vi "graphics.vi"() -> ()   [LabVIEW 2018]
panel:
  in  "Tab Control":enum32{"CONTROLLER", "TEMP", "PRESSURE"}(tab)
  out "FEED WATER\nMOTOR AMPS\nPHASE A":dbl(knob) scale=0.0..10.0
  in  "V in":dbl
  out "Vout 2":dbl
  out "Vin":u8(slide) scale=0.0..100.0
  out "Vout":u8(slide) scale=0.0..20.0
  out "FEED WATER \nMOTOR AMPS \nPHASE B":dbl(knob) scale=0.0..10.0
  in  "DEG F":dbl
  out "DEG C":dbl
  out "DEG\nF":u8(slide) scale=0.0..100.0
  out "DEG\nC":u8(slide) scale=0.0..100.0
  out "FEED WATER \nMOTOR AMPS\nPHASE C":dbl(knob) scale=0.0..10.0
  in  "lbs/sq in":dbl
  out "mm Hg":dbl
  out "lb/sq\nin":u8(slide) scale=0.0..100.0
  out "mm\nHg":u8(slide) scale=0.0..100.0
  in  "stop":bool
  # "BOILER #1 FEED\nWATER CONTROL"
  # "FIC 1000\nFEED WATER\nCONTROLLER"
  # "FIC 1000\nFEED WATER\nTEMP"
  # "FIC 1000\nFEED WATER\nPRESSURE"
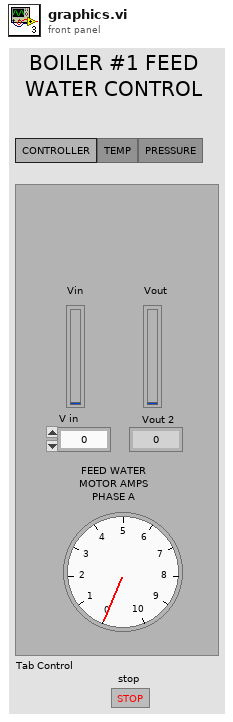
[diagram p1: front panel]
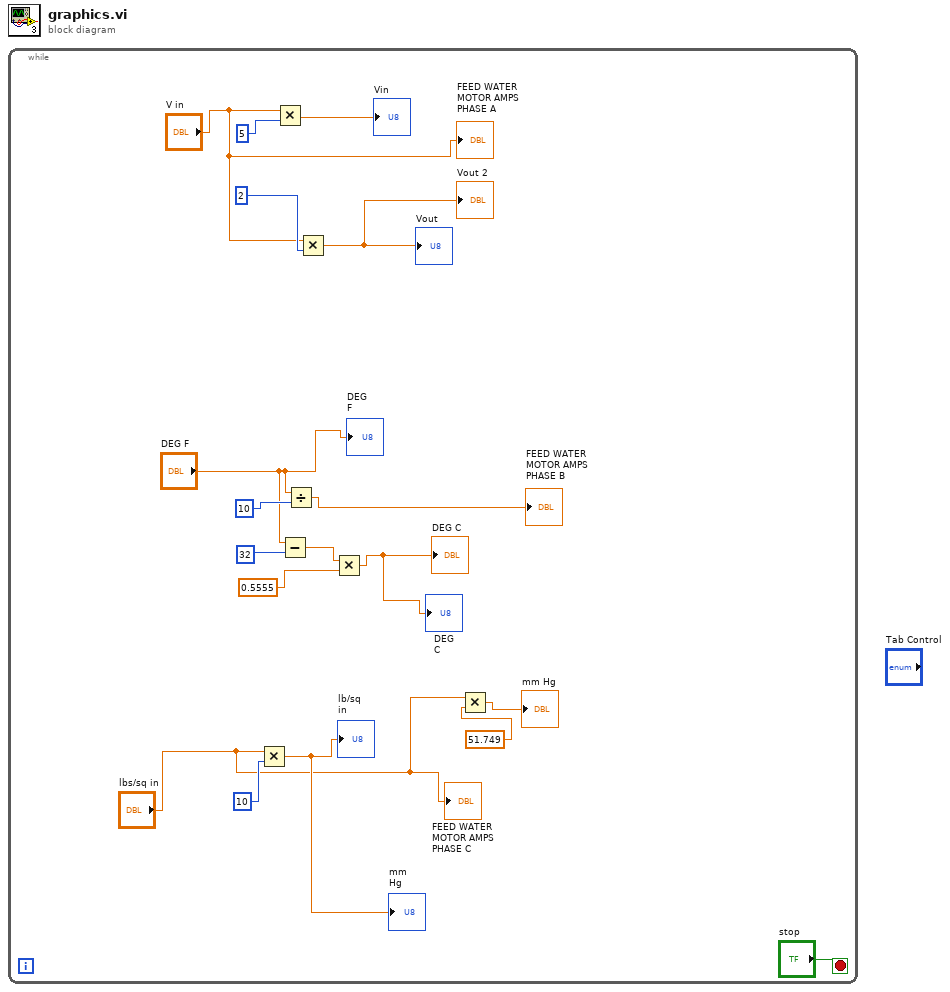
[diagram p0: block diagram]
diagram:
  n1 = while {
    stop <- "stop" stop-if-true
    n2 = Multiply(x="lbs/sq in", y=10) -> (x*y=→"lb/sq\nin" →"mm\nHg":dbl)
    n3 = Multiply(x="V in", y=5) -> (x*y=→"Vin":dbl)
    n4 = Subtract(x="DEG F", y=32) -> (x-y=w12:dbl)
    n5 = Divide(x="DEG F", y=10) -> (x/y=→"FEED WATER \nMOTOR AMPS \nPHASE B":dbl)
    n6 = Multiply(x="V in", y=2) -> (x*y=→"Vout 2" →"Vout":dbl)
    n7 = Multiply(x=w12, y=0.5555) -> (x*y=→"DEG C" →"DEG\nC":dbl)
    n8 = Multiply(x="lbs/sq in", y=51.749) -> (x*y=→"mm Hg":dbl)
    "FEED WATER\nMOTOR AMPS\nPHASE A" <- "V in"
    "FEED WATER \nMOTOR AMPS\nPHASE C" <- "lbs/sq in"
    "DEG\nF" <- "DEG F"
  }
